vi "NML Cont Acquire and Store.vi"() -> ()   [LabVIEW 2025]
doc: "I. Description:\nThis example demonstrates how to acquire a continuous amount of data (Waveform) using the DAQ device's internal clock.\n\nII. Instructions for Running:\n1. Create empty task\n2. Create an analog input voltage channel.\n3. Set the rate for the sample clock. Additionally, define the sample mode to be continuous.\n4. Call the Start VI to start the acquisition.\n5. Read the waveform data in a loop until the user hits the stop button or an error occurs.\nNote: This example reads data from one or more channels and returns an array of data. Use the Index Array function to access an individual channel of data.\n6. Stop the analog input task\n7. Call the Clear Task VI to clear the Task.\n8. Use the popup dialog box to display an error if any.\n\nIV. I/O Connections Overview:\nMake sure your signal input terminal matches the Physical Channel I/O Control. For further connection information, refer to your hardware reference manual.\nAuthor: Scott Hannahs <sth@magnet.fsu.edu>\n\nThis software is licensed for use under the “MIT License\"\nCopyright (c) 2025 Scott Hannahs, sth@sth@magnet.sthnet.net\n\nPermission is hereby granted, free of charge, to any person obtaining a copy of this software and associated documentation files (the \"Software\"), to deal in the Software without restriction, including without limitation the rights to use, copy, modify, merge, publish, distribute, sublicense, and/or sell copies of the Software, and to permit persons to whom the Software is furnished to do so, subject to the following conditions: The above copyright notice and this permission notice shall be included in all copies or substantial portions of the Software.\n\nTHE SOFTWARE IS PROVIDED \"AS IS\", WITHOUT WARRANTY OF ANY KIND, EXPRESS OR IMPLIED, INCLUDING BUT NOT LIMITED TO THE WARRANTIES OF MERCHANTABILITY, FITNESS FOR A PARTICULAR PURPOSE AND NONINFRINGEMENT. IN NO EVENT SHALL THE AUTHORS OR COPYRIGHT HOLDERS BE LIABLE FOR ANY CLAIM, DAMAGES OR OTHER LIABILITY, WHETHER IN AN ACTION OF CONTRACT, TORT OR OTHERWISE, ARISING FROM, OUT OF OR IN CONNECTION WITH THE SOFTWARE OR THE USE OR OTHER DEALINGS IN THE SOFTWARE."
uses:
  <vilib>/Utility/error.llb/DialogType.ctl
  <vilib>/_DAQmxBase/Internals/DAQmxBase Create Channel (AI-Voltage-Basic).vi
  <vilib>/_DAQmxBase/Internals/DAQmxBase Timing (Sample Clock).vi
  <vilib>/_DAQmxBase/Internals/DAQmxBase Read (Analog 2D DBL NChan NSamp).vi
panel:
  out "Scan Backlog":u32
  out "Display Iteration":i32
  out "Store Iteration":i32
  out "Acq Iteration":i32
  in  "Filename":string="Test"
  in  "Physical Channel":tag="Dev1/ai0:7"
  in  "Samples to Read":i32=1700
  in  "Minimum Value":dbl=-0.001 format="%.3f"
  in  "Maximum Value":dbl=0.001 format="%.3f"
  in  "stop":bool
  in  "Sample Rate":dbl=120000.0 caption="Sample Rate (Hz)"
  out "Measurement":dbl[][](graph)
  # "For instructions, select Help>>Show Context Help"
  # "Channel Parameters"
  # "Timing Parameters"
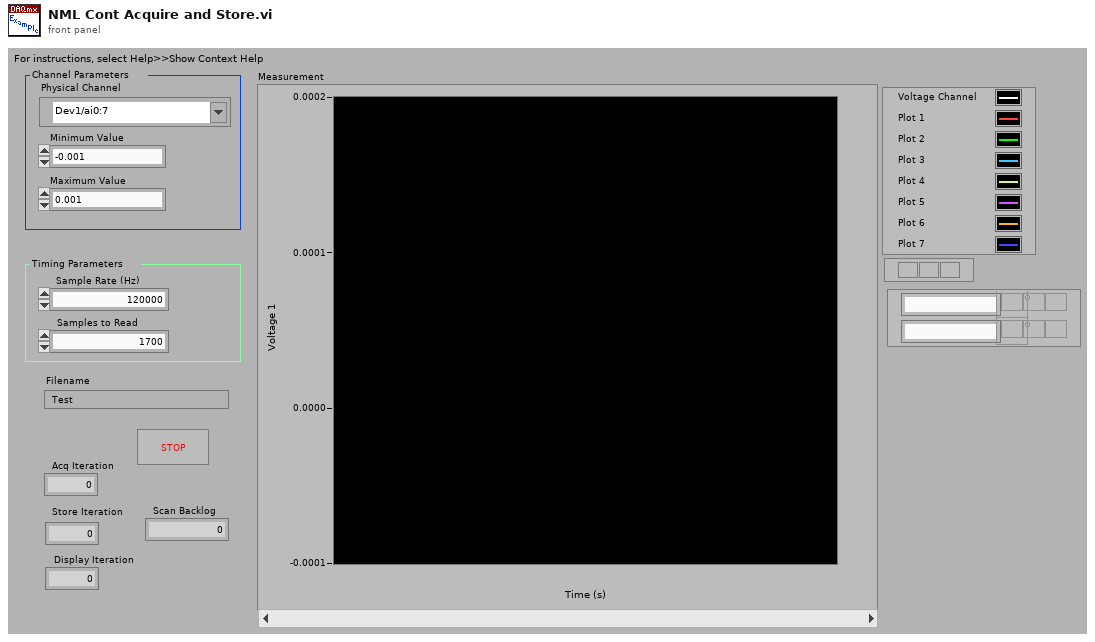
[diagram p1: front panel]
types:
  T1 = typedef "DialogType.ctl" = u16
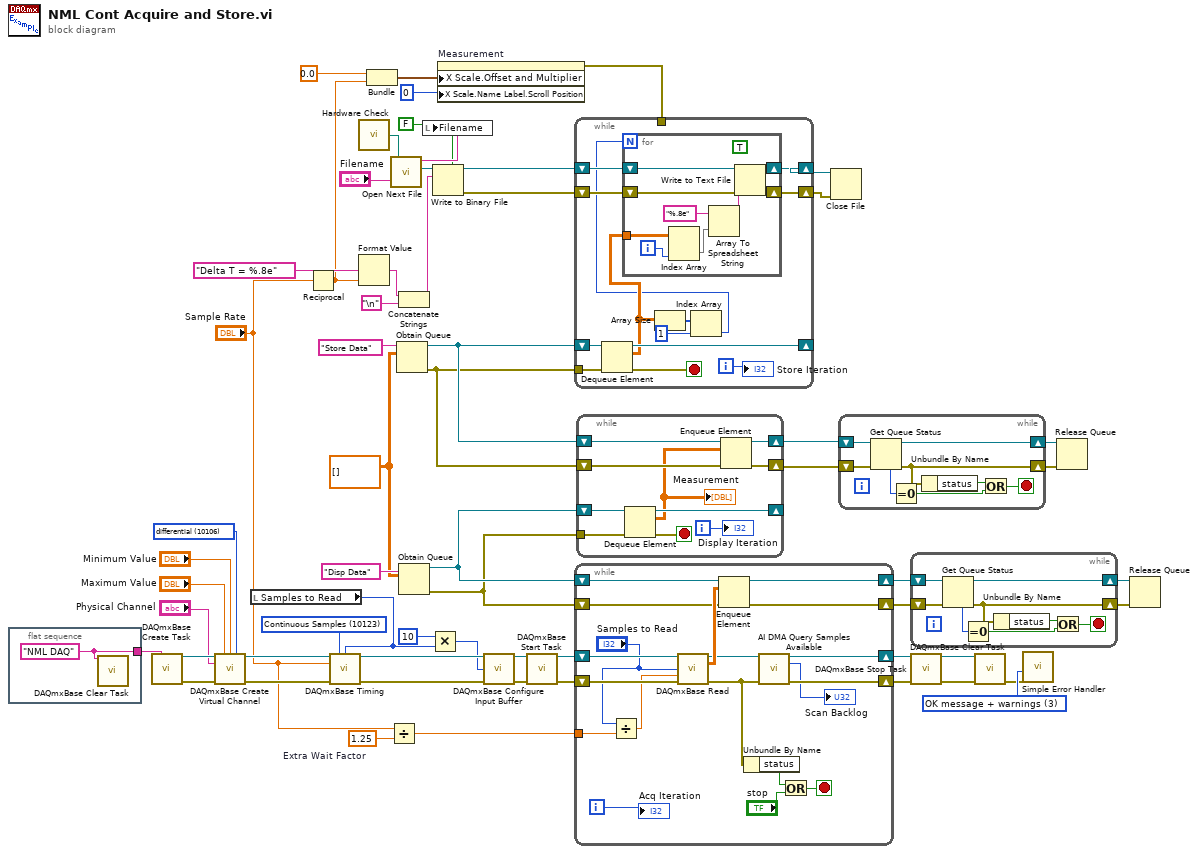
[diagram p0: block diagram]
diagram:
  w1 = 1.25  # Extra Wait Factor
  w18 = dbl[][] [] ("data")
  w43 = 10106 items=["default"=-1, "differential"=10106, "RSE"=10083, "NRSE"=10078] ("input terminal configuration")
  w60 = T1 3 items=["no dialog", "OK message", "continue or stop message", "OK message + warnings", "continue/stop + warnings"] ("type of dialog (OK msg:1)")
  w47 = 10123 items=["Finite Samples"=10178, "Continuous Samples"=10123] ("sample mode")
  n1 = flat-sequence {
    tunnel: [w61] -> w8
    frame #0 {
      w61 = "NML DAQ" ("new task name")
      n2 = call <vilib>:"DAQmxBase Clear Task.vi"("task in"=w61) -> ()  [unwired: 14 in, 1 out]
    }
  }
  n3 = call <vilib>:"DAQmxBase Create Task.vi"("new task name"=w8) -> ("task out"=w58:refnum<k21>, "error out"=w59:errorcluster)  [unwired: 13 in]
  n4 = call-poly <vilib>:"DAQmxBase Create Virtual Channel.vi"("task in"=w58, "maximum value"="Maximum Value", "minimum value"="Minimum Value", "input terminal configuration"=w43, "physical channels"="Physical Channel", "error in"=w59) -> ("task out"=w56:refnum<k21>, "error out"=w57:errorcluster)  [unwired: 8 in]
  n5 = local read "Samples to Read"() -> (w6:i32)
  n6 = Reciprocal(x="Sample Rate") -> (1/x=w33:dbl)
  n7 = call-poly <vilib>:"DAQmxBase Timing.vi"("task/channels in"=w56, "sample mode"=w47, "samples per channel"=w6, "rate"="Sample Rate", "error in"=w57) -> ("task out"=w54:refnum<k21>, "error out"=w55:errorcluster)  [unwired: 9 in]
  n8 = call "Hardware Check.vi"() -> ("Data Directory Path"=w40:path)  [unwired: 1 in, 2 out]
  n9 = Format Value(format string="Delta T = %.8e" ("format"), value (0)=w33) -> (output string=w39:string)  [unwired: 1 in]
  n10 = Bundle(0.0, w33) -> (w34:cluster{dbl, dbl})  [unwired: 1 in]
  n11 = Divide(x="Sample Rate", y=w1) -> (x/y=w2:dbl)
  n12 = call "Open Next File.vi"("Input File Pattern"="Filename", "Dir Path"=w40) -> ("File Ref Num"=w36:refnum<file>, "Output File Name"=w41:string)  [unwired: 1 in, 2 out]
  n13 = Obtain Queue(name (unnamed)="Store Data", element data type=w18) -> (queue out=w17:refnum<queue>, error out=w10:errorcluster)  [unwired: 3 in, 1 out]
  n14 = Concatenate Strings(w39, "\n") -> (w35:string)
  n15 = Obtain Queue(name (unnamed)="Disp Data", element data type=w18) -> (queue out=w16:refnum<queue>, error out=w11:errorcluster)  [unwired: 3 in, 1 out]
  n16 = local write "Filename"(w41) -> ()
  n17 = Multiply(x=u32 10, y=w6) -> (x*y=w5:u32)
  n18 = Write to Binary File(file (use dialog)=w36, data=w35, 5:FALSE ("prepend array or string size? (T)")) -> (refnum out=w30:refnum<file>, error out=w29:errorcluster)  [unwired: 3 in, 1 out]
  n19 = property on="Measurement" class="WFChart (strict)"("X Scale.Offset and Multiplier"=w34, "X Scale.Name Label.Scroll Position"=u32 0) -> (error out=w24:errorcluster)  [unwired: 2 in, 1 out]
  n20 = call <vilib>:"DAQmxBase Configure Input Buffer.vi"("task/channels in"=w54, "buffer size (in samples per channel)"=w5) -> ("task out"=w7:refnum<k21>)  [unwired: 12 in, 1 out]
  n21 = call <vilib>:"DAQmxBase Start Task.vi"("task/channels in"=w7, "error in"=w55) -> ("task out"=w53:refnum<k21>, "error out"=w27:errorcluster)  [unwired: 12 in]
  n22 = while {
    shift-right: [w72] -> w26
    shift-left: w30 -> [w73]
    shift-right: [w71] -> w25
    shift-left: w29 -> [w74]
    tunnel: w24 -> [_]
    shift-right: [w68] -> _
    shift-left: w17 -> [w70]
    tunnel: w10 -> [w67]
    i -> [w66]
    stop <- w69 stop-if-true
    n23 = Dequeue Element(queue=w70, error in (no error)=w67) -> (queue out=w68:refnum<queue>, element=w65:dbl[][], error out=w69:errorcluster)  [unwired: 1 in, 1 out]
    n24 = Array Size(array=w65) -> (size(s)=w64:i32[])
    n25 = Index Array(array=w64, index=1) -> (element=w63:i32)
    n26 = for {
      N: w63 -> [_]
      shift-right: [w81] -> w72
      shift-left: w73 -> [w82]
      shift-right: [w80] -> w71
      shift-left: w74 -> [w83]
      tunnel: w65 -> [w77]
      i -> [w75]
      (unwired) TRUE ("convert eol (F)")
      n27 = Index Array(array=w77, index (col)=w75) -> (element=w76:dbl[])  [unwired: 1 in]
      n28 = Array To Spreadsheet String(array=w76, 3:"%.8e" ("format")) -> (spreadsheet string=w78:string)  [unwired: 1 in]
      n29 = Write to Text File(file (use dialog)=w82, text=w78, error in=w83) -> (refnum out=w81:refnum<file>, error out=w80:errorcluster)  [unwired: 1 in, 1 out]
    }
    "Store Iteration" <- w66
  }
  n30 = while {
    shift-right: [w93] -> w20
    shift-left: w11 -> [w92]
    shift-right: [w94] -> w21
    shift-left: w16 -> [w95]
    tunnel: w2 -> [w84]
    shift-right: [w89] -> w52
    shift-left: w53 -> [w101]
    shift-right: [w90] -> w48
    shift-left: w27 -> [w102]
    i -> [w97]
    stop <- w98 stop-if-true
    n31 = Divide(x="Samples to Read", y=w84) -> (x/y=w86:dbl)
    n32 = call-poly <vilib>:"DAQmxBase Read.vi"("task/channels in"=w101, "number of samples per channel"="Samples to Read", "timeout"=w86, "error in"=w102) -> ("task out"=w88:refnum<k21>, "data"=w96:dbl[][], "error out"=w91:errorcluster)  [unwired: 9 in]
    n33 = Enqueue Element(queue=w95, element=w96, error in (no error)=w92) -> (queue out=w94:refnum<queue>, error out=w93:errorcluster)  [unwired: 1 in, 1 out]
    n34 = Unbundle By Name(w91) -> ("status"=w99:bool)
    n35 = call "AI DMA Query Samples Available.vi"("task in"=w88, "error in"=w91) -> ("task out"=w89:refnum<k21>, "samples per chan available"=→"Scan Backlog":u32, "error out"=w90:errorcluster)  [unwired: 11 in]
    n36 = Or(x=w99, y="stop") -> (x .or. y?=w98:bool)
    "Acq Iteration" <- w97
  }
  n37 = while {
    shift-right: [w110] -> w13
    shift-left: w17 -> [w107]
    shift-right: [w109] -> w12
    shift-left: w10 -> [w108]
    shift-right: [w111] -> _
    shift-left: w16 -> [w112]
    tunnel: w11 -> [w104]
    i -> [w103]
    stop <- w105 stop-if-true
    n38 = Dequeue Element(queue=w112, error in (no error)=w104) -> (queue out=w111:refnum<queue>, element=w106:dbl[][], error out=w105:errorcluster)  [unwired: 1 in, 1 out]
    "Measurement" <- w106
    n39 = Enqueue Element(queue=w107, element=w106, error in (no error)=w108) -> (queue out=w110:refnum<queue>, error out=w109:errorcluster)  [unwired: 1 in, 1 out]
    "Display Iteration" <- w103
  }
  n40 = Close File(refnum=w26, error in=w25) -> ()  [unwired: 2 out]
  n41 = while {
    shift-right: [w116] -> w15
    shift-left: w12 -> [w119]
    shift-right: [w118] -> w14
    shift-left: w13 -> [w120]
    stop <- w117 stop-if-true
    n42 = Get Queue Status(queue=w120, error in (no error)=w119) -> (queue out=w118:refnum<queue>, error out=w116:errorcluster, # elements in queue=w115:i32)  [unwired: 1 in, 5 out]
    n43 = Equal To 0?(x=w115) -> (x = 0?=w113:bool)
    n44 = Unbundle By Name(w116) -> ("status"=w114:bool)
    n45 = Or(x=w114, y=w113) -> (x .or. y?=w117:bool)
  }
  n46 = while {
    shift-right: [w124] -> w22
    shift-left: w20 -> [w127]
    shift-right: [w126] -> w23
    shift-left: w21 -> [w128]
    stop <- w125 stop-if-true
    n47 = Get Queue Status(queue=w128, error in (no error)=w127) -> (queue out=w126:refnum<queue>, error out=w124:errorcluster, # elements in queue=w123:i32)  [unwired: 1 in, 5 out]
    n48 = Equal To 0?(x=w123) -> (x = 0?=w121:bool)
    n49 = Unbundle By Name(w124) -> ("status"=w122:bool)
    n50 = Or(x=w122, y=w121) -> (x .or. y?=w125:bool)
  }
  n51 = call <vilib>:"DAQmxBase Stop Task.vi"("task/channels in"=w52, "error in"=w48) -> ("task out"=w50:refnum<k21>, "error out"=w51:errorcluster)  [unwired: 12 in]
  n52 = call <vilib>:"DAQmxBase Clear Task.vi"("task in"=w50, "error in"=w51) -> ("error out"=w49:errorcluster)  [unwired: 13 in]
  n53 = call <vilib>:"Simple Error Handler.vi"("type of dialog (OK msg:1)"=w60, "error in (no error)"=w49) -> ()  [unwired: 3 in, 5 out]
  n54 = Release Queue(queue=w14, error in (no error)=w15) -> ()  [unwired: 1 in, 3 out]
  n55 = Release Queue(queue=w23, error in (no error)=w22) -> ()  [unwired: 1 in, 3 out]
